vi "获取种子坐标.vi"() -> ()   [LabVIEW 2023]
panel:
  out "Center of Mass":cluster{"X":dbl, "Y":dbl}
  in  "Center of Mass 2":cluster{"X":dbl, "Y":dbl}
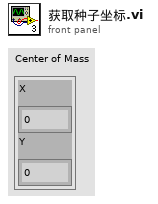
[diagram p1: front panel]
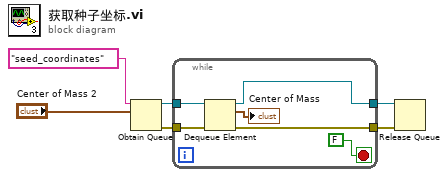
[diagram p0: block diagram]
diagram:
  n1 = Obtain Queue(name (unnamed)="seed_coordinates" ("名称（未命名）"), element data type="Center of Mass 2") -> (queue out=w5:refnum<queue>, error out=w4:errorcluster)  [unwired: 3 in, 1 out]
  n2 = while {
    tunnel: w5 -> [w12]
    tunnel: w4 -> [w11]
    tunnel: [w10] -> w3
    tunnel: [w9] -> w2
    stop <- FALSE stop-if-true
    n3 = Dequeue Element(queue=w12, error in (no error)=w11) -> (queue out=w9:refnum<queue>, element=→"Center of Mass":cluster{"X":dbl, "Y":dbl}, error out=w10:errorcluster)  [unwired: 1 in, 1 out]
  }
  n4 = Release Queue(queue=w2, error in (no error)=w3) -> ()  [unwired: 1 in, 3 out]
